vi "BRig_Host__Loop_Consumer_RunState__getThresholds.vi"(8 "threshold_2":u16, 9 "threshold_1":u16, 10 "input_idx":i32[](array[numeric]), 11 "input_dataTS":u16[][](array[numeric])) -> (0 "output_threshold_2":u16, 1 "output_threshold_1":u16, 2 "output_haveThresholds":bool)   [LabVIEW 2014]
uses:
  <vilib>/Utility/file.llb/Write To Spreadsheet File (DBL).vi
panel:
  out "standard output":string
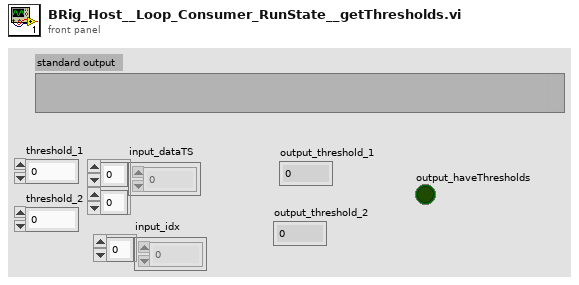
[diagram p1: front panel]
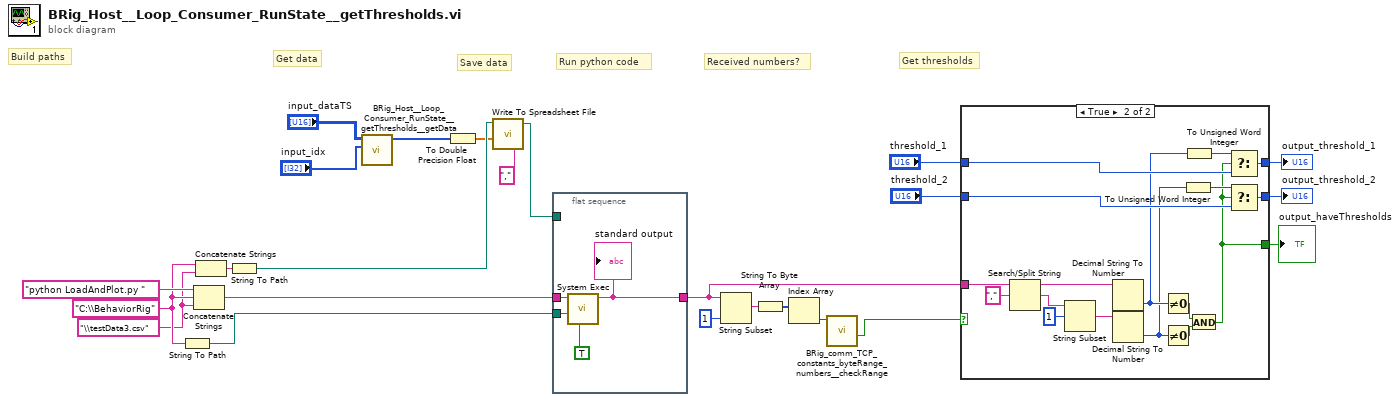
[diagram p0: block diagram]
diagram:
  w9 = "C:\\BehaviorRig"
  w8 = "\\testData3.csv"
  # "Get thresholds"
  # "Run python code"
  # "Save data"
  # "Get data"
  # "Build paths"
  # "Received numbers?"
  n1 = String To Path(string=w9) -> (path=w13:path)
  n2 = Concatenate Strings("python LoadAndPlot.py " ("command line"), w9, w8) -> (w10:string)
  n3 = Concatenate Strings(w9, w8) -> (w7:string)
  n4 = String To Path(string=w7) -> (path=w12:path)
  n5 = call "BRig_Host__Loop_Consumer_RunState__getThresholds__getData.vi"("input_idx"="input_idx", "input_dataTS"="input_dataTS") -> ("output_data"=w4:u16[])  [unwired: 9 in]
  n6 = To Double Precision Float(number=w4) -> (double precision float=w2:dbl[])
  n7 = call-poly <vilib>:"Write To Spreadsheet File.vi"("delimiter (\\t)"="," ("delimiter (\\t)"), "1D data"=w2, "file path (dialog if empty)"=w12) -> ("new file path (Not A Path if cancelled)"=w11:path)  [unwired: 5 in]
  n8 = flat-sequence {
    tunnel: [w27] -> w20
    tunnel: w13 -> [w26]
    tunnel: w10 -> [w25]
    tunnel: w11 -> [_]
    frame #0 {
      n9 = call <vilib>:"System Exec.vi"("run minimized? (F)"=TRUE, "working directory"=w26, "command line"=w25) -> ("standard output"=w27:string)  [unwired: 5 in, 3 out]
      "standard output" <- w27
    }
  }
  n10 = String Subset(string=w20, length (rest)=1 ("length (rest)")) -> (substring=w23:string)  [unwired: 1 in]
  n11 = String To Byte Array(string=w23) -> (unsigned byte array=w22:u8[])
  n12 = Index Array(array=w22) -> (element=w21:u8)  [unwired: 1 in]
  n13 = call "BRig_comm_TCP_constants_byteRange_numbers__checkRange.vi"("input_byte"=w21) -> ("output_numbers_num"=w6:bool)  [unwired: 8 in, 2 out]
  n14 = case shown="True" w6 {
    tunnel: w20 -> [_ w47]
    tunnel: "threshold_1" -> [w30 w38]
    tunnel: [w30 w39] -> w16
    tunnel: "threshold_2" -> [w29 w36]
    tunnel: [w29 w37] -> w15
    tunnel: [_ w31] -> w1
    frame False {
    }
    frame True {
      n15 = Search/Split String(string=w47, search string/char (-)=",") -> (substring before match=w42:string, match + rest of string=w45:string)  [unwired: 1 in, 1 out]
      n16 = String Subset(string=w45, offset (0)=1) -> (substring=w43:string)  [unwired: 1 in]
      n17 = Decimal String To Number(string=w42) -> (number=w35:i32)  [unwired: 2 in, 1 out]
      n18 = Decimal String To Number(string=w43) -> (number=w34:i32)  [unwired: 2 in, 1 out]
      n19 = Not Equal To 0?(x=w35) -> (x != 0?=w40:bool)
      n20 = Not Equal To 0?(x=w34) -> (x != 0?=w41:bool)
      n21 = To Unsigned Word Integer(number=w34) -> (unsigned 16bit integer=w33:u16)
      n22 = To Unsigned Word Integer(number=w35) -> (unsigned 16bit integer=w32:u16)
      n23 = And(x=w40, y=w41) -> (x .and. y?=w31:bool)
      n24 = Select(t=w32, s=w31, f=w38) -> (s? t:f=w39:u16)
      n25 = Select(t=w33, s=w31, f=w36) -> (s? t:f=w37:u16)
    }
  }
  "output_threshold_1" <- w16
  "output_threshold_2" <- w15
  "output_haveThresholds" <- w1
